vi "RTS Macro Determine Power Period.vi"(1 "Refrigeration Core Stats Input":T1 {"Average Compressor Cycle Time (Min)" format="%0.2f"; "Average Compressor Power (W)" format="%0.2f"; "Power Start Time (sec)" format="%<%H:%M:%S>t"; "Power End time (sec)" format="%<%H:%M:%S>t"; "Average Defrost Power (W)" format="%0.2f"}, 2 "Refrigeration Full Data":T2, 3 "Error In":errorcluster) -> (7 "Full Time":dbl[](array[numeric]), 8 "Refrigeration Core Stats Output":T1 {"Average Compressor Cycle Time (Min)" format="%0.2f"; "Average Compressor Power (W)" format="%0.2f"; "Power Start Time (sec)" format="%<%H:%M:%S>t"; "Power End time (sec)" format="%<%H:%M:%S>t"; "Average Defrost Power (W)" format="%0.2f"}, 10 "Error Out":errorcluster)   [LabVIEW 2016]
uses:
  Type Definitions/RTS Macro Full Data.ctl
  Type Definitions/RTS Macro Refrigeration Core Stats.ctl
panel:
  out "Wh Full":dbl[](array[numeric])
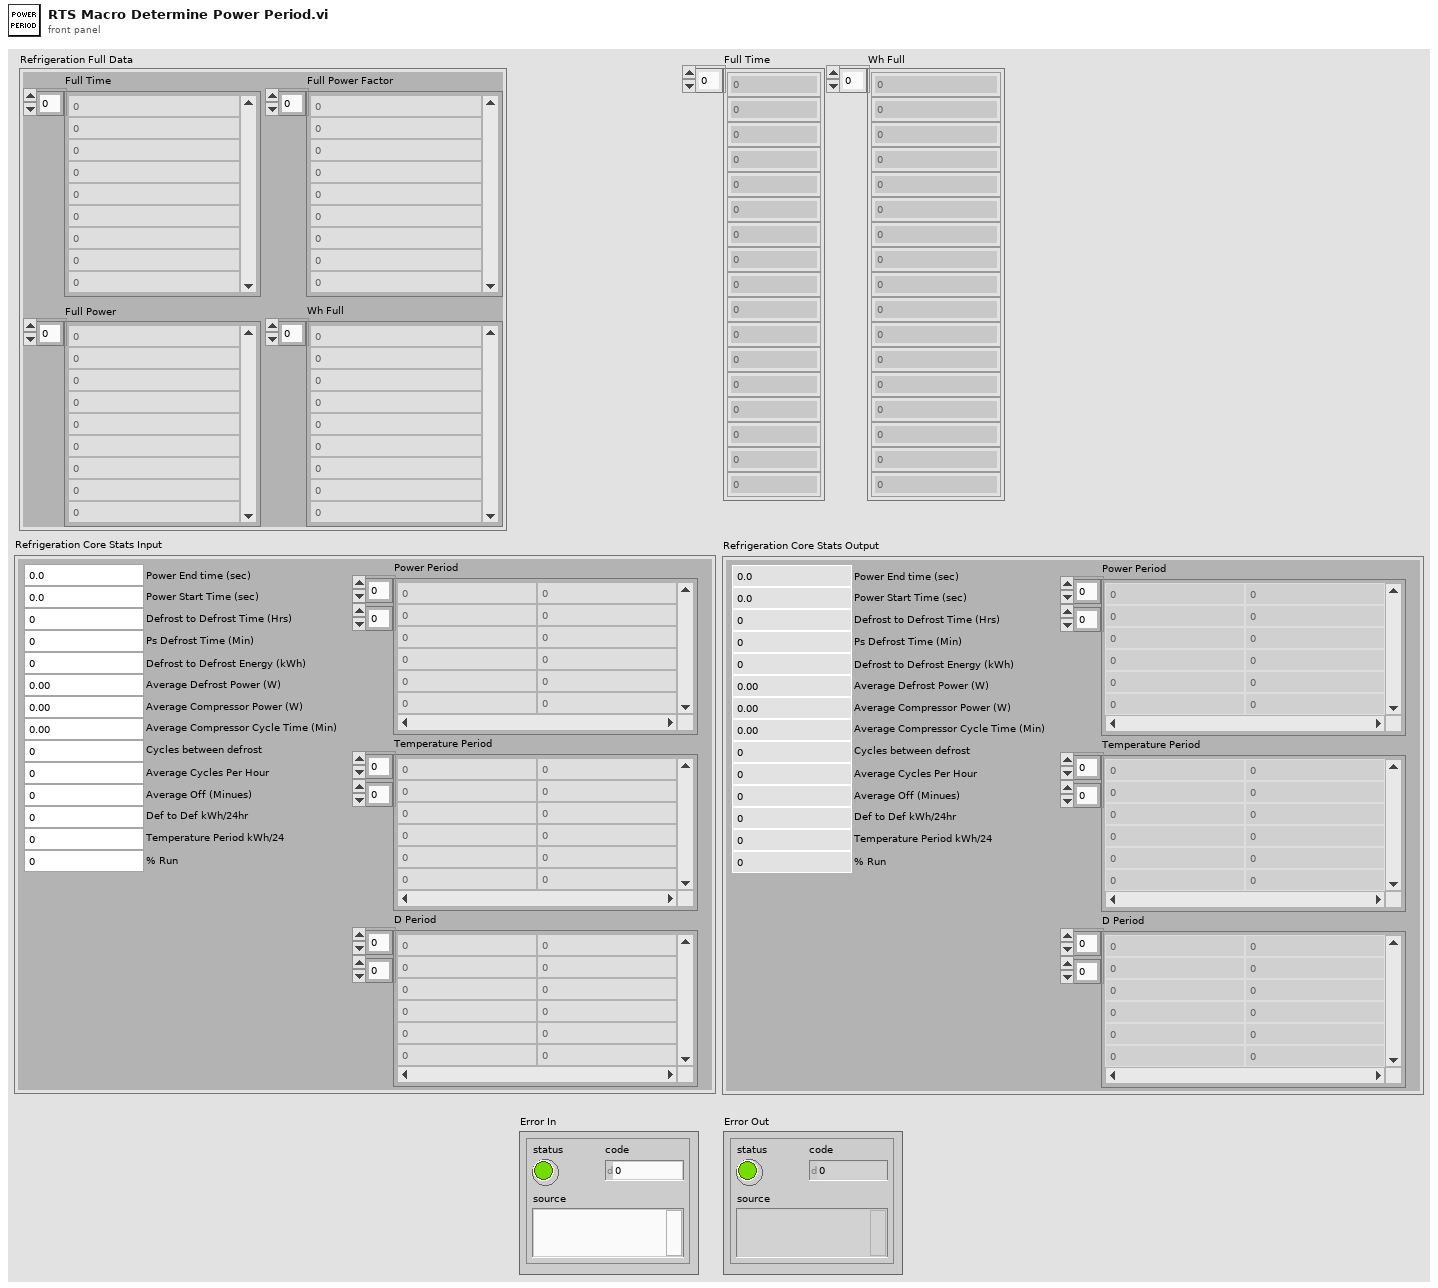
[diagram p1: front panel]
types:
  T1 = typedef "RTS Macro Refrigeration Core Stats.ctl" = cluster{"Average Defrost Power (W)":dbl, "Power End time (sec)":dbl, "Power Start Time (sec)":dbl, "Defrost to Defrost Time (Hrs)":dbl, "Ps Defrost Time (Min)":dbl, "Defrost to Defrost Energy (kWh)":dbl, "Average Compressor Power (W)":dbl, "Average Compressor Cycle Time (Min)":dbl, "Power Period":dbl[][], "Cycles between defrost":i32, "Average Cycles Per Hour":dbl, "Average Off (Minues)":dbl, "Def to Def kWh/24hr":dbl, "Temperature Period kWh/24":dbl, "% Run":dbl, "Temperature Period":dbl[][], "D Period":dbl[][]}
  T2 = typedef "RTS Macro Full Data.ctl" = cluster{"Full Time":dbl[], "Full Power Factor":dbl[], "Full Power":dbl[], "Wh Full":dbl[]}
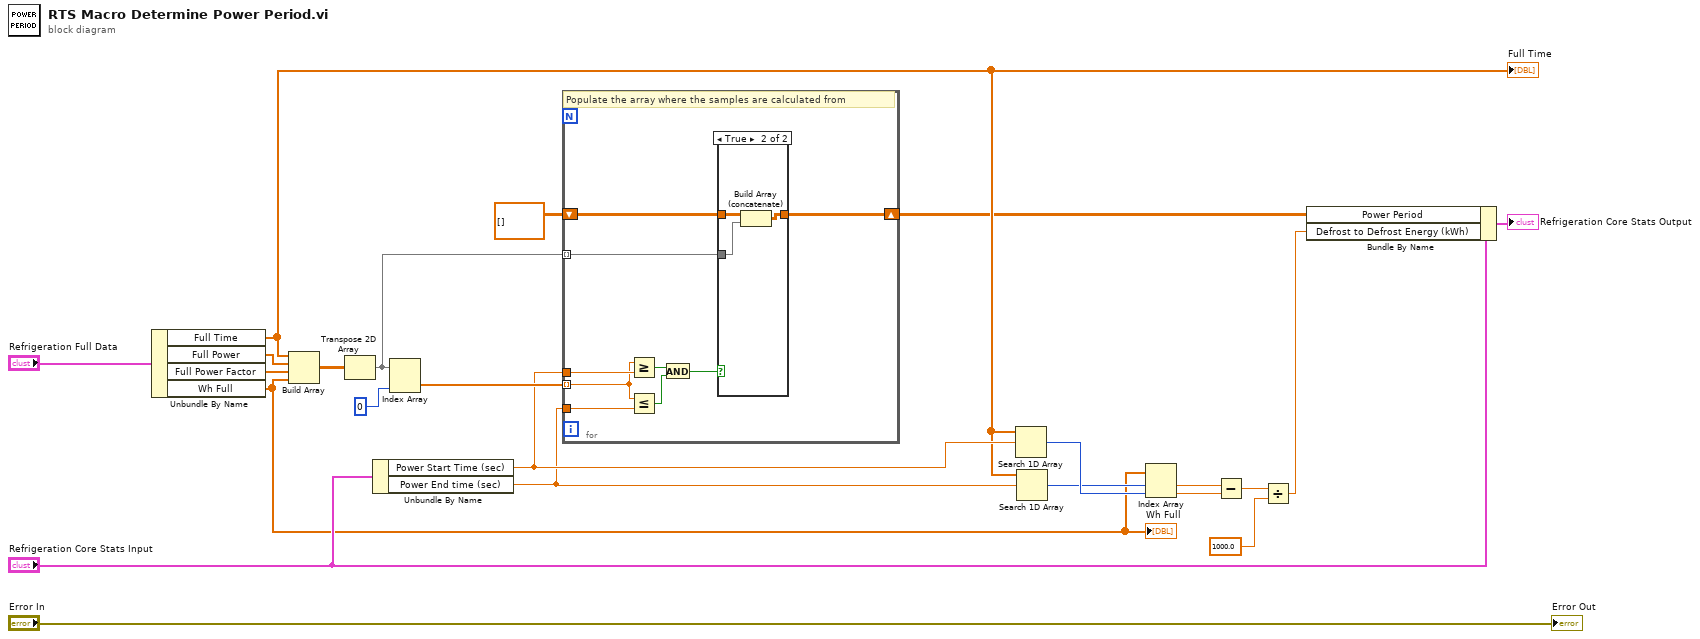
[diagram p0: block diagram]
diagram:
  n1 = Unbundle By Name("Refrigeration Full Data") -> ("Full Time"=w5:dbl[], "Full Power"=w21:dbl[], "Full Power Factor"=w23:dbl[], "Wh Full"=w3:dbl[])
  "Wh Full" <- w3
  "Full Time" <- w5
  n2 = Build Array(w5, w21, w23, w3) -> (w16:dbl[][])
  n3 = Transpose 2D Array(2D array=w16) -> (transposed array=w20:dbl[][])
  n4 = Unbundle By Name("Refrigeration Core Stats Input") -> ("Power Start Time (sec)"=w7:dbl, "Power End time (sec)"=w6:dbl)
  n5 = Index Array(array=w20, index (col)=0 ("disabled index (col)")) -> (element=w18:dbl[])  [unwired: 1 in]
  n6 = for {
    tunnel: w18 -> [w31] mode=indexing
    tunnel: w7 -> [w32]
    tunnel: w6 -> [w30]
    tunnel: w20 -> [w26] mode=indexing
    shift-right: [w24] -> w4
    shift-left: dbl[][] [] -> [w25]
    # "Populate the array where the samples are calculated from"
    n7 = Greater Or Equal?(x=w31, y=w32) -> (x >= y?=w29:bool)
    n8 = Less Or Equal?(x=w31, y=w30) -> (x <= y?=w28:bool)
    n9 = And(x=w29, y=w28) -> (x .and. y?=w27:bool)
    n10 = case shown="True" w27 {
      tunnel: w26 -> [_ w35]
      tunnel: w25 -> [w33 w36]
      tunnel: [w33 w34] -> w24
      frame False {
      }
      frame True {
        n11 = Build Array (concatenate)(w36, w35) -> (w34:dbl[][])
      }
    }
  }
  n12 = Search 1D Array(1D array=w5, element=w7) -> (index of element=w9:i32)  [unwired: 1 in]
  n13 = Search 1D Array(1D array=w5, element=w6) -> (index of element=w8:i32)  [unwired: 1 in]
  n14 = Index Array(array=w3, index #1=w8, index #2=w9) -> (element #1=w11:dbl, element #2=w10:dbl)
  n15 = Subtract(x=w11, y=w10) -> (x-y=w12:dbl)
  n16 = Divide(x=w12, y=1000.0) -> (x/y=w2:dbl)
  n17 = Bundle By Name(cluster="Refrigeration Core Stats Input", "Power Period"=w4, "Defrost to Defrost Energy (kWh)"=w2) -> (→"Refrigeration Core Stats Output":T1)
  "Error Out" <- "Error In"
